vi "读取.vi"(8 "error in (no error)":errorcluster caption="错误输入（无错误）", 10 "PLC指令":T1={"变量类型"=2, "PLC地址"="0", "16位/32位"=0, "写入数据(写入时有效)"=""} {"16位/32位" items=["16bit", "32bit"]; "变量类型" items=["X", "Y", "M", "D"]}, 11 "PLC设置":T2={"端口选择"="COM3", "波特率"=9600, "校检"=2, "数据位"=7} {"数据位" items=["7"=7, "8"=8]; "校检" items=["无", "偶", "奇"]; "波特率" items=["9600"=9600, "19200"=19200, "115200"=115200]}) -> (0 "error out":errorcluster caption="错误输出", 2 "读取成功":bool)   [LabVIEW 2015, in "PLC.lvlib"]
uses:
  PLC.lvlib
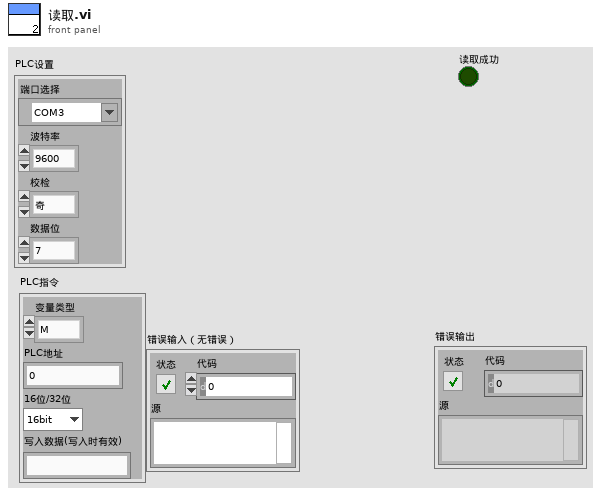
[diagram p1: front panel]
types:
  T1 = typedef "PLC.lvlib/PLC指令.ctl" = cluster{"变量类型":u32, "PLC地址":string, "16位/32位":u32, "写入数据(写入时有效)":string}
  T2 = typedef "PLC.lvlib/PLC设置.ctl" = cluster{"端口选择":refnum<visa-resource-name>, "波特率":u32, "校检":u32, "数据位":u32}
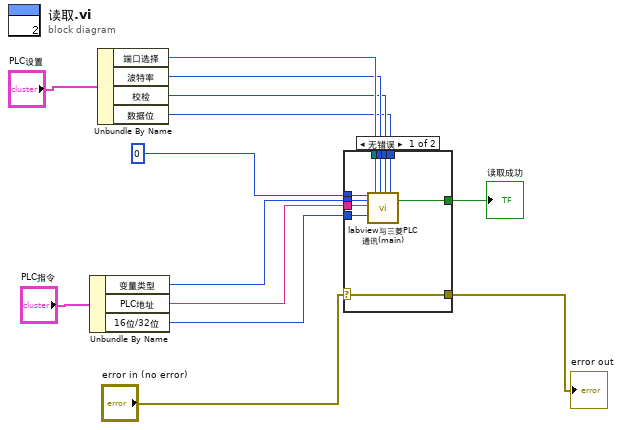
[diagram p0: block diagram]
diagram:
  n1 = Unbundle By Name("PLC指令") -> ("变量类型"=w6:u32, "PLC地址"=w5:string, "16位/32位"=w4:u32)
  n2 = Unbundle By Name("PLC设置") -> ("端口选择"=w12:refnum<visa-resource-name>, "波特率"=w10:u32, "校检"=w9:u32, "数据位"=w8:u32)
  n3 = case shown="无错误" "error in (no error)" {
    selector: "error in (no error)" -> [w14 w24]
    tunnel: w12 -> [w23 _]
    tunnel: i16 0 ("读取=0写入=1") -> [w22 _]
    tunnel: w10 -> [w21 _]
    tunnel: w9 -> [w20 _]
    tunnel: w8 -> [w19 _]
    tunnel: w6 -> [w18 _]
    tunnel: w5 -> [w17 _]
    tunnel: w4 -> [w16 _]
    tunnel: [w15 _] -> w3
    tunnel: [w14 w24] -> w1
    frame No Error {
      n4 = call "labview与三菱PLC通讯(main).vi"("读取=0写入=1"=w22, "变量类型"=w18, "PLC地址"=w17, "16位/32位"=w16, "端口选择"=w23, "波特率"=w21, "校检"=w20, "数据位"=w19) -> ("读取成功"=w15:bool)  [unwired: 9 in, 2 out]
    }
    frame Error {
    }
  }
  "读取成功" <- w3
  "error out" <- w1
